vi "test-trapezoid-profile-cont-under-vel-change.vi"() -> ()   [LabVIEW 2019]
uses:
  <vilib>/Rock Robotics/WPI/ThirdParty/JAS_Junk/TrajLib/TRAPEZOID_PROFILE_STATE.ctl
  <vilib>/Rock Robotics/WPI/ThirdParty/JAS_Junk/TrajLib/TRAPEZOID_PROFILE.ctl
  <vilib>/Rock Robotics/WPI/ThirdParty/JAS_Junk/TrajLib/TRAPEZOID_PROFILE_CONSTRAINT.ctl
  <vilib>/Rock Robotics/WPI/ThirdParty/JAS_Junk/TrajLib/TrapProfile_Direct.vi
  <vilib>/Rock Robotics/WPI/ThirdParty/JAS_Junk/TrajLib/TrapProfile_ShouldFlipAcceleration.vi
  <vilib>/Rock Robotics/WPI/ThirdParty/JAS_Junk/TrajLib/Trajectory_Library.lvlib
panel:
  out "TRAPEZOID_PROFILE":T1 {"Goal"."Velocity" format="%16_6e"; "Goal"."Position" format="%16_6e"; "Initial"."Velocity" format="%16_6e"; "Initial"."Position" format="%16_6e"; "Constraints"."MaxAcceleration" format="%16_6e"; "Constraints"."MaxVelocity" format="%16_6e"; "EndDecel" format="%16_6e"; "EndFullSpeed" format="%16_6e"; "EndAccel" format="%16_6e"}
  out "State":T3 {"Velocity" format="%16_6e"; "Position" format="%16_6e"}
  out "Waveform Chart":T4(graph)
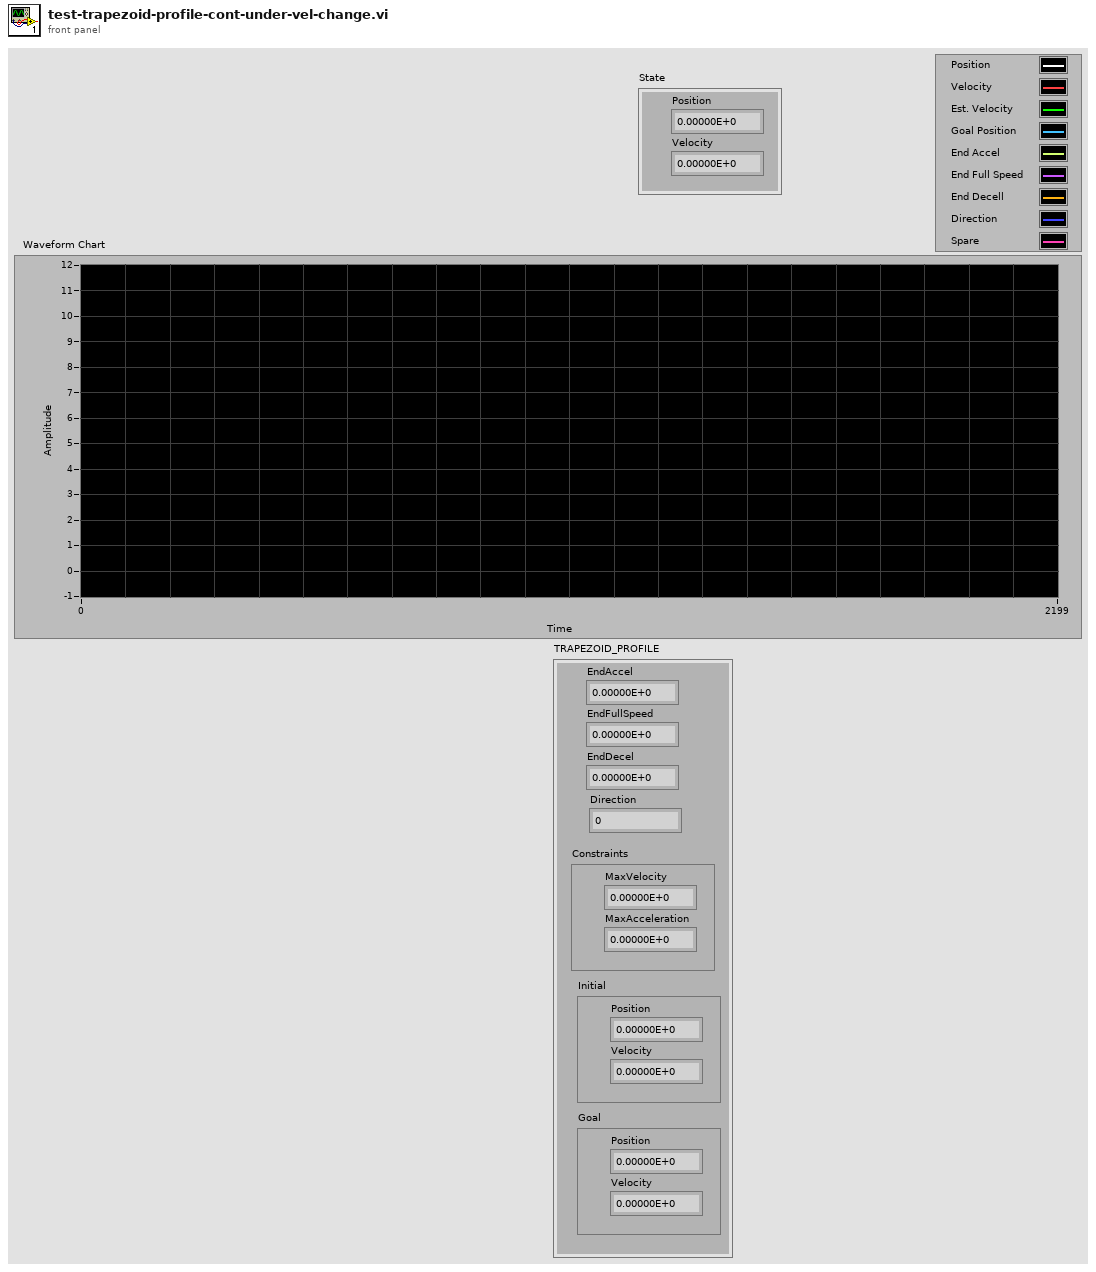
[diagram p1: front panel]
types:
  T1 = typedef "Trajectory_Library.lvlib/TRAPEZOID_PROFILE.ctl" = cluster{"EndAccel":dbl, "EndFullSpeed":dbl, "EndDecel":dbl, "Direction":i32, "Constraints":T2, "Initial":T3, "Goal":T3}
  T2 = typedef "Trajectory_Library.lvlib/TRAPEZOID_PROFILE_CONSTRAINT.ctl" = cluster{"MaxVelocity":dbl, "MaxAcceleration":dbl}
  T3 = typedef "Trajectory_Library.lvlib/TRAPEZOID_PROFILE_STATE.ctl" = cluster{"Position":dbl, "Velocity":dbl}
  T4 = cluster{"Position":dbl, "Velocity":dbl, dbl, "Position":dbl, "EndAccel":dbl, "EndFullSpeed":dbl, "EndDecel":dbl, "Direction":i32, "Position":dbl}
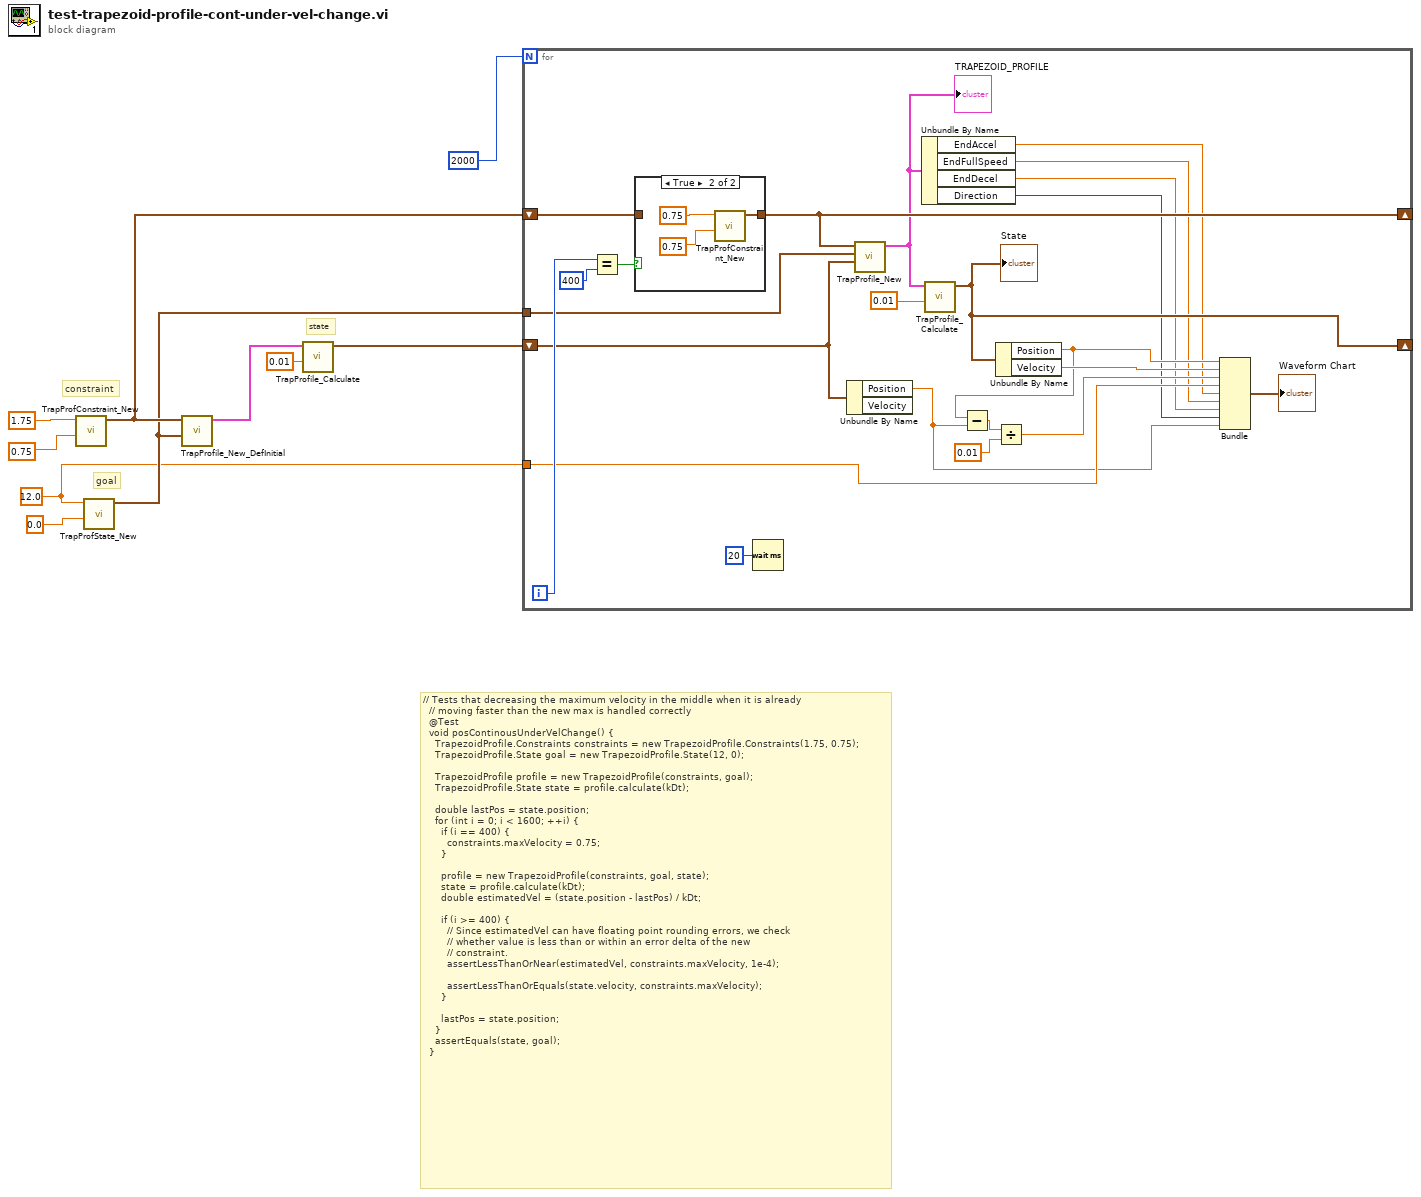
[diagram p0: block diagram]
diagram:
  w1 = 12.0 ("Position")
  # "// Tests that decreasing the maximum velocity in the middle when it is already\n  // moving faster than the new max is handled correctly\n  @Test\n  void posContinousUnderVelChange() {\n    TrapezoidProfile.Constraints constraints = new TrapezoidProfile.Constraints(1.75, 0.75);\n    TrapezoidProfile.State goal = new TrapezoidProfile.State(12, 0);\n\n    TrapezoidProfile profile = new TrapezoidProfile(constraints, goal);\n    TrapezoidProfile.State state = profile.calculate(kDt);\n\n    double lastPos = state.position;\n    for (int i = 0; i < 1600; ++i) {\n      if (i == 400) {\n        constraints.maxVelocity = 0.75;\n      }\n\n      profile = new TrapezoidProfile(constraints, goal, state);\n      state = profile.calculate(kDt);\n      double estimatedVel = (state.position - lastPos) / kDt;\n\n      if (i >= 400) {\n        // Since estimatedVel can have floating point rounding errors, we check\n        // whether value is less than or within an error delta of the new\n        // constraint.\n        assertLessThanOrNear(estimatedVel, constraints.maxVelocity, 1e-4);\n\n        assertLessThanOrEquals(state.velocity, constraints.maxVelocity);\n      }\n\n      lastPos = state.position;\n    }\n    assertEquals(state, goal);\n  }"
  # "goal"
  # "state"
  # "constraint"
  n1 = call <vilib>:"TrapProfConstraint_New.vi"("Max Accel"=0.75, "Max Speed (M/S)"=1.75) -> ("TRAPEZOID_PROFILE_CONSTRAINT"=w3:T2)  [unwired: 9 in]
  n2 = call <vilib>:"TrapProfState_New.vi"("Velocity"=0.0, "Position"=w1) -> ("TRAPEZOID_PROFILE_STATE"=w2:T3)  [unwired: 9 in]
  n3 = call <vilib>:"TrapProfile_New_DefInitial.vi"("Goal"=w2, "Constraints"=w3) -> ("TRAPEZOID_PROFILE"=w6:T1)  [unwired: 9 in]
  n4 = call <vilib>:"TrapProfile_Calculate.vi"("Time"=0.01, "TRAPEZOID_PROFILE"=w6) -> ("State"=w4:T3)  [unwired: 9 in]
  n5 = for {
    N: 2000 -> [_]
    shift-right: [w18] -> _
    shift-left: w4 -> [w23]
    shift-right: [w26] -> _
    shift-left: w3 -> [w27]
    tunnel: w2 -> [w25]
    tunnel: w1 -> [w17]
    i -> [w29]
    n6 = Equal?(x=w29, y=400) -> (x = y?=w30:bool)
    n7 = case shown="True" w30 {
      tunnel: [w34 w35] -> w26
      tunnel: w27 -> [w34 _]
      frame False {
      }
      frame True {
        n8 = call <vilib>:"TrapProfConstraint_New.vi"("Max Accel"=0.75, "Max Speed (M/S)"=0.75) -> ("TRAPEZOID_PROFILE_CONSTRAINT"=w35:T2)  [unwired: 9 in]
      }
    }
    n9 = Wait (ms)(milliseconds to wait=u32 20) -> ()  [unwired: 1 out]
    n10 = Unbundle By Name(w23) -> ("Position"=w11:dbl)  [unwired: 1 out]
    n11 = call <vilib>:"TrapProfile_New.vi"("Initial"=w23, "Goal"=w25, "Constraints"=w26) -> ("TRAPEZOID_PROFILE"=w16:T1)  [unwired: 8 in]
    "TRAPEZOID_PROFILE" <- w16
    n12 = Unbundle By Name(w16) -> ("EndAccel"=w15:dbl, "EndFullSpeed"=w14:dbl, "EndDecel"=w13:dbl, "Direction"=w12:i32)
    n13 = call <vilib>:"TrapProfile_Calculate.vi"("Time"=0.01, "TRAPEZOID_PROFILE"=w16) -> ("State"=w18:T3)  [unwired: 9 in]
    "State" <- w18
    n14 = Unbundle By Name(w18) -> ("Position"=w22:dbl, "Velocity"=w31:dbl)
    n15 = Subtract(x=w22, y=w11) -> (x-y=w21:dbl)
    n16 = Divide(x=w21, y=0.01) -> (x/y=w19:dbl)
    n17 = Bundle("Position"=w22, "Velocity"=w31, w19, "Position"=w17, "EndAccel"=w15, "EndFullSpeed"=w14, "EndDecel"=w13, "Direction"=w12, "Position"=w11) -> (→"Waveform Chart":T4)  [unwired: 1 in]
  }
